vi "Hold Dataset.vi"(8 "error in (no error)":errorcluster, 9 "Group ID":string, 10 "Data In":dbl[](array[numeric]), 11 "DAO Actions":T1) -> (0 "error out":errorcluster, 2 "Data Out":dbl[](array[numeric]))   [LabVIEW 2013]
uses:
  Data Access Objects/Metadata/DAO Actions.ctl
panel:
  out "Dataset":variant
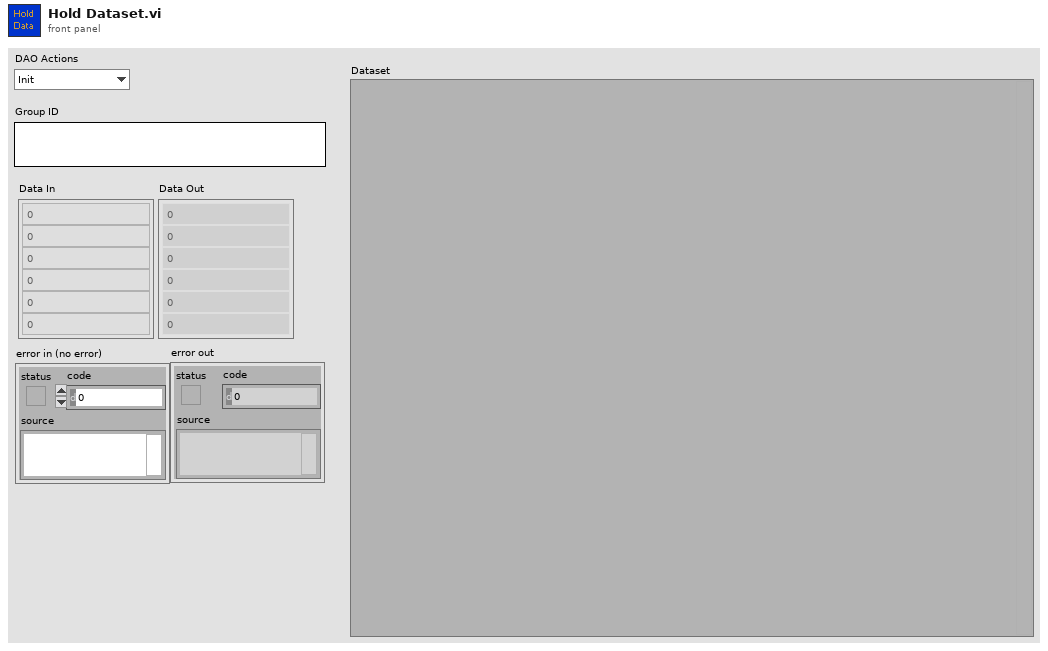
[diagram p1: front panel]
types:
  T1 = typedef "DAO Actions.ctl" = enum16{"Init", "Get", "Set"}
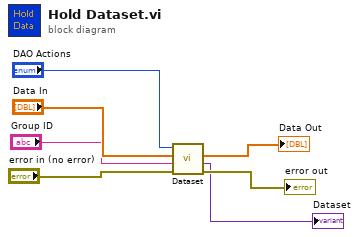
[diagram p0: block diagram]
diagram:
  n1 = call "Dataset.vi"("error in (no error)"="error in (no error)", "Group ID"="Group ID", "Data In"="Data In", "DAO Actions"="DAO Actions") -> ("error out"=→"error out":errorcluster, "Dataset"=→"Dataset":variant, "Data Out"=→"Data Out":dbl[])  [unwired: 5 in]
